vi "setPinValYldrm.vi"(2 "YLDRMErrorInp":errorcluster, 3 "val":u8, 4 "pin":u8, 5 "YLDRMPortInp":refnum<visa-resource-name>) -> (0 "YLDRMErrorOut":errorcluster, 1 "YLDRMPortOut":refnum<visa-resource-name>)   [LabVIEW 2015]
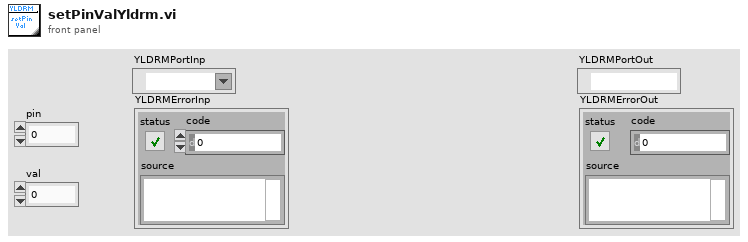
[diagram p1: front panel]
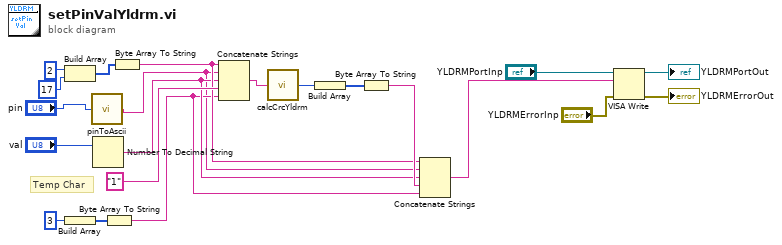
[diagram p0: block diagram]
diagram:
  # "Temp Char"
  n1 = Build Array(2, 17) -> (w19:i32[])
  n2 = Build Array(3) -> (w15:i32[])
  n3 = call "pinToAscii.vi"("inp"="pin") -> ("out"=w2:string)
  n4 = Number To Decimal String(number="val") -> (decimal integer string=w4:string)  [unwired: 1 in]
  n5 = Byte Array To String(unsigned byte array=w15) -> (string=w3:string)
  n6 = Byte Array To String(unsigned byte array=w19) -> (string=w5:string)
  n7 = Concatenate Strings(w5, w2, w4, "1", w3) -> (w6:string)
  n8 = call "calcCrcYldrm.vi"("inpStr"=w6) -> ("crcVal"=w14:u8)
  n9 = Build Array(w14) -> (w13:u8[])
  n10 = Byte Array To String(unsigned byte array=w13) -> (string=w8:string)
  n11 = Concatenate Strings(w5, w2, w4, w8, w3) -> (w7:string)
  n12 = VISA Write(VISA resource name="YLDRMPortInp", write buffer=w7, error in (no error)="YLDRMErrorInp") -> (VISA resource name out=→"YLDRMPortOut":refnum<visa-resource-name>, error out=→"YLDRMErrorOut":errorcluster)  [unwired: 1 out]
